vi "FPGA_target_execute_function.vi"(0 "tick_count_in":u32, 2 "data_in":T1, 4 "set_stop_output_in":bool, 5 "input_data_in":u8, 7 "stop_request":bool, 8 "fifo_empty_in":bool, 9 "C0_data":T2, 11 "C1_data":T2) -> (10 "set_output":bool, 12 "read_fifo":bool, 13 "stop":bool, 14 "tick_count_out":u32, 16 "data_dup":T1, 17 "fifo_empty_out":bool, 18 "set_stop_output_out":bool, 19 "input_data_out":u8)   [LabVIEW 2014]
doc: "executes a command (time, wait, jump, stop)"
uses:
  FPGA_32BitPattern_data_type.ctl
  FPGA_cmd_data_type.ctl
  <vilib>/rvi/eio/common/nirviEmuTemplateMethod_errors.vi
  <vilib>/eio/EIONode/EIONode.xnode
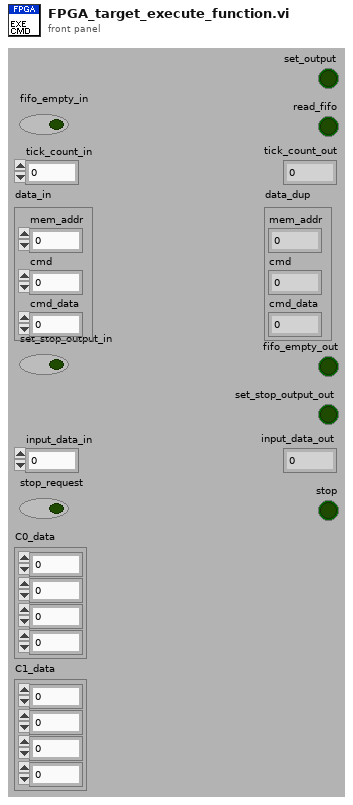
[diagram p1: front panel]
types:
  T1 = typedef "FPGA_cmd_data_type.ctl" = cluster{"mem_addr":u32, "cmd":u8, "cmd_data":u32}
  T2 = typedef "FPGA_32BitPattern_data_type.ctl" = cluster{"port0":u8, "port1":u8, "port2":u8, "port3":u8}
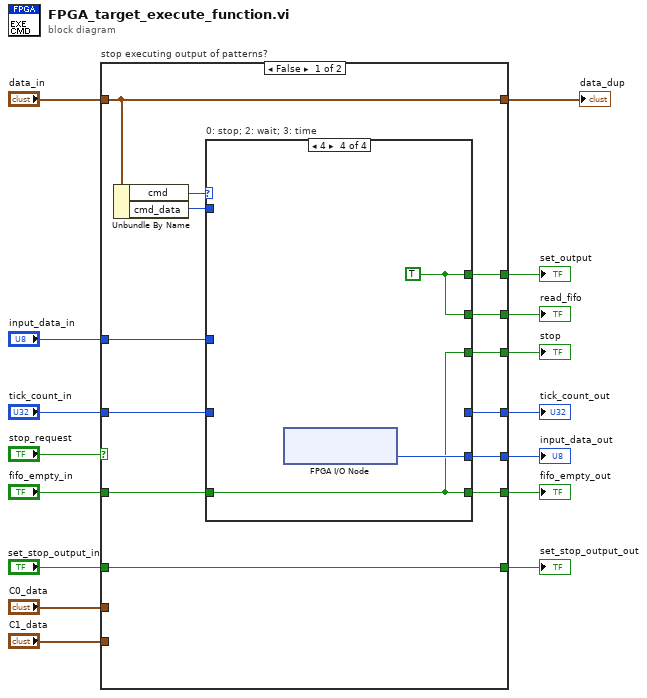
[diagram p0: block diagram]
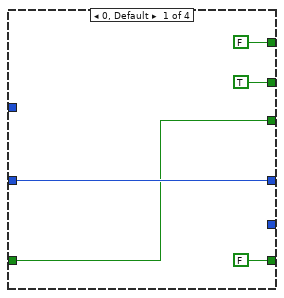
[diagram p2: hidden frame]
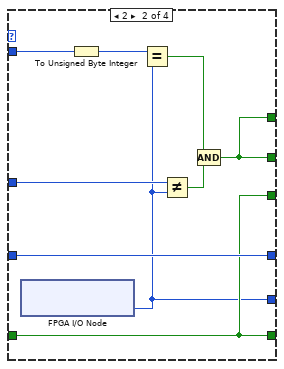
[diagram p3: hidden frame]
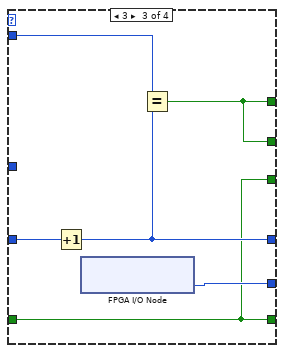
[diagram p4: hidden frame]
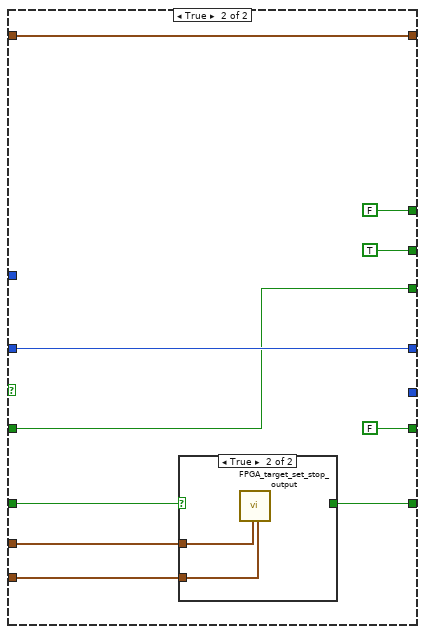
[diagram p5: hidden frame]
diagram:
  n1 = case "stop executing output of patterns?" shown="False" "stop_request" {
    tunnel: "tick_count_in" -> [w29 w61]
    tunnel: [w28 FALSE] -> w15
    tunnel: [w27 w61] -> w14
    tunnel: [w26 w54] -> w13
    tunnel: "fifo_empty_in" -> [w22 w54]
    tunnel: [w17 TRUE] -> w10
    tunnel: [w25 _] -> w9
    tunnel: "input_data_in" -> [w24 _]
    tunnel: "set_stop_output_in" -> [w23 w59]
    tunnel: "C0_data" -> [_ w58]
    tunnel: "C1_data" -> [_ w57]
    tunnel: [w23 w56] -> w4
    tunnel: "data_in" -> [w21 w55]
    tunnel: [w21 w55] -> w2
    tunnel: [w18 FALSE ("fifo_empty_in")] -> w1
    frame False {
      n2 = Unbundle By Name(w21) -> ("cmd"=w20:u8, "cmd_data"=w19:u32)
      n3 = case "0: stop; 2: wait; 3: time" shown="4" w20 {
        tunnel: w19 -> [_ w40 w49 _]
        tunnel: w29 -> [w34 w43 w47 _]
        tunnel: [FALSE w37 w44 w50] -> w28
        tunnel: [w34 w43 w46 _] -> w27
        tunnel: [w32 w38 w45 w51] -> w26
        tunnel: [_ w35 w48 w52] -> w25
        tunnel: w24 -> [_ w36 _ _]
        tunnel: w22 -> [w32 w38 w45 w51]
        tunnel: [FALSE ("fifo_empty_in") w38 w45 w51] -> w18
        tunnel: [TRUE ("fifo_empty") w37 w44 w50] -> w17
        frame 0, Default {
        }
        frame 2 {
          n4 = xnode ("FPGA I/O Node")() -> ("TriggerIn_0-7"=w35:u8)  [unwired: 1 in, 1 out]
          n5 = To Unsigned Byte Integer(number=w40) -> (unsigned 8bit integer=w41:u8)
          n6 = Equal?(x=w41, y=w35) -> (x = y?=w42:bool)
          n7 = Not Equal?(x=w36, y=w35) -> (x != y?=w39:bool)
          n8 = Compound Arithmetic op=AND(w42, w39) -> (w37:bool)
        }
        frame 3 {
          n9 = Increment(x=w47) -> (x+1=w46:u32)
          n10 = xnode ("FPGA I/O Node")() -> ("TriggerIn_0-7"=w48:u8)  [unwired: 1 in, 1 out]
          n11 = Equal?(x=w49, y=w46) -> (x = y?=w44:bool)
        }
        frame 4 {
          w50 = TRUE
          n12 = xnode ("FPGA I/O Node")() -> ("TriggerIn_0-7"=w52:u8)  [unwired: 1 in, 1 out]
        }
      }
    }
    frame True {
      n13 = case shown="True" w59 {
        selector: w59 -> [w63 _]
        tunnel: w58 -> [_ w65]
        tunnel: w57 -> [_ w64]
        tunnel: [w63 _] -> w56
        frame False {
        }
        frame True {
          n14 = call "FPGA_target_set_stop_output.vi"("connector0_data"=w65, "connector1_data"=w64) -> ()  [unwired: 18 in]
        }
      }
    }
  }
  "set_output" <- w15
  "tick_count_out" <- w14
  "stop" <- w13
  "read_fifo" <- w10
  "input_data_out" <- w9
  "set_stop_output_out" <- w4
  "data_dup" <- w2
  "fifo_empty_out" <- w1
